vi "GCS3_Finish_Motion_Error.vi"(0 "System no.":i32=1 min=1 max=4 step=1, 2 "Axis (ContainerUnit)":string, 3 "PID controller (FunctionUnit)":string, 4 "Original PID values":string[](array[string]), 5 "error in":errorcluster) -> (19 "error out":errorcluster)   [LabVIEW 2026]
doc: "Prepares a PI GCS 3.0 system for motion error by setting the PID parameters to zero. This is only a sample. Do not use in production code.\n\nCompatibility: This sample requires a PI GCS 3.0 controller."
panel:
  # "Finish the motion error of a PI GCS 3.0 system by restoring the PID parameters.\nThis is only a sample. Do not use in production code.\n\nCompatibility: This sample requires a PI GCS 3.0 controller."
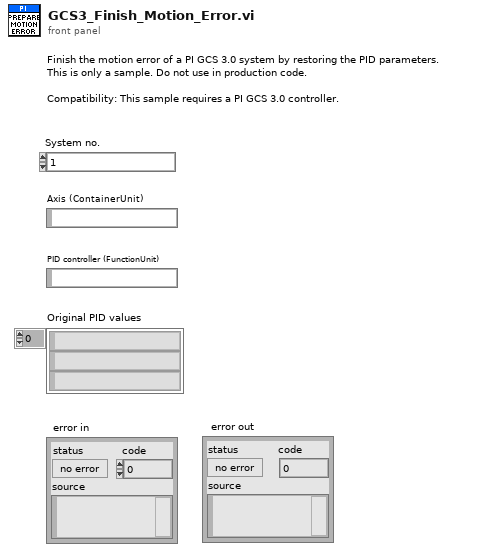
[diagram p1: front panel]
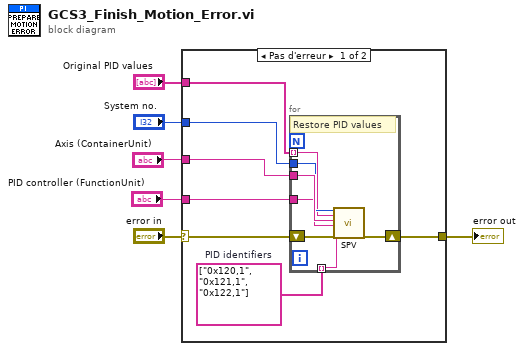
[diagram p0: block diagram]
diagram:
  n1 = case shown="Pas d'erreur" "error in" {
    selector: "error in" -> [w7 w21]
    tunnel: "PID controller (FunctionUnit)" -> [w13 _]
    tunnel: "Axis (ContainerUnit)" -> [w12 _]
    tunnel: [w11 w21] -> w6
    tunnel: "System no." -> [w9 _]
    tunnel: "Original PID values" -> [w8 _]
    frame No Error {
      w10 = string[] ["0x120,1", "0x121,1", "0x122,1"]  # PID identifiers
      n2 = for {
        tunnel: w10 -> [w17] mode=indexing
        shift-right: [w20] -> w11
        shift-left: w7 -> [w14]
        tunnel: w12 -> [w19]
        tunnel: w13 -> [w18]
        tunnel: w9 -> [w16]
        tunnel: w8 -> [w15] mode=indexing
        # "Restore PID values"
        n3 = call "SPV.vi"("System no."=w16, "ParameterSet"=w19, 3:w18, 4:w17, "error in"=w14, 6:w15) -> ("error out"=w20:errorcluster)  [unwired: 13 in]
      }
    }
    frame Error {
    }
  }
  "error out" <- w6
